vi "Translate Rectangle.vi"(10 "offset":cluster{"x":i16, "y":i16}, 11 "Rectangle in":T1) -> (3 "Rectangle out":T1)   [LabVIEW 2021, in "Picture Pixel Fonts.lvlib"]
uses:
  <vilib>/LabVIEW Icon API/Pixel Fonts/Picture Pixel Fonts.lvlib
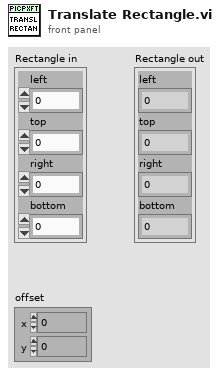
[diagram p1: front panel]
types:
  T1 = cluster{"left":i16, "top":i16, "right":i16, "bottom":i16}
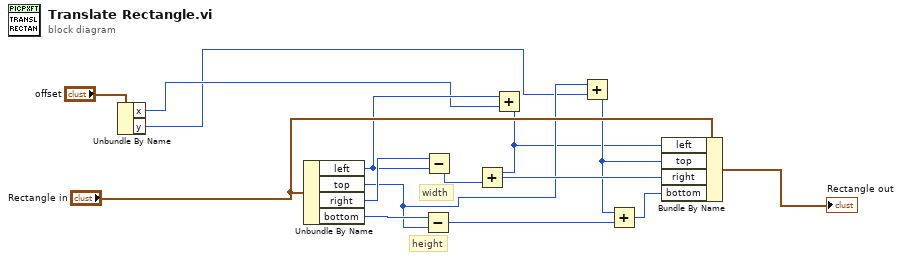
[diagram p0: block diagram]
diagram:
  # "width"
  # "height"
  n1 = Unbundle By Name("offset") -> ("x"=w5:i16, "y"=w3:i16)
  n2 = Unbundle By Name("Rectangle in") -> ("left"=w6:i16, "top"=w4:i16, "right"=w11:i16, "bottom"=w8:i16)
  n3 = Subtract(x=w8, y=w4) -> (x-y=w10:i16)
  n4 = Subtract(x=w11, y=w6) -> (x-y=w13:i16)
  n5 = Add(x=w6, y=w5) -> (x+y=w1:i16)
  n6 = Add(x=w1, y=w13) -> (x+y=w15:i16)
  n7 = Add(x=w4, y=w3) -> (x+y=w2:i16)
  n8 = Add(x=w2, y=w10) -> (x+y=w12:i16)
  n9 = Bundle By Name(cluster="Rectangle in", "left"=w1, "top"=w2, "right"=w15, "bottom"=w12) -> (→"Rectangle out":T1)
